vi "Berechnung Limit mbar.vi"(0 "Volumen in mm³":dbl, 1 "t2":timestamp, 2 "t1":timestamp, 7 "p1":sgl, 9 "T2 in C°":sgl, 11 "T1 in C°":sgl, 12 "Fluss in l/min":sgl) -> (4 "Limit in mbar":sgl format="%#.9f", 8 "p2":dbl)   [LabVIEW 2020, in "EPA 1065.lvlib" / "Dichtheitstest 1065-345.lvlib"]
uses:
  Dichtheitstest 1065-345.lvlib
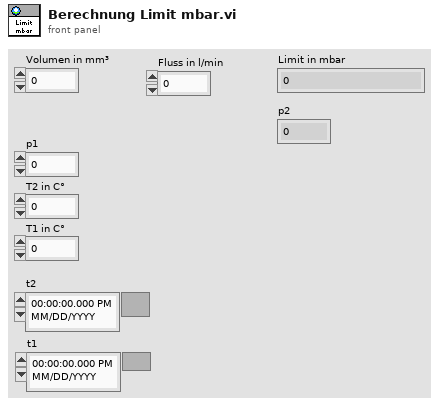
[diagram p1: front panel]
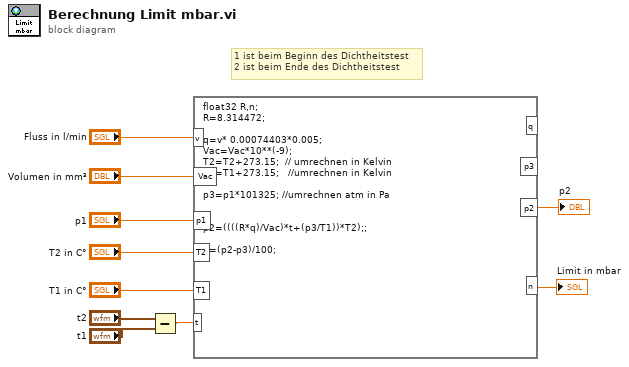
[diagram p0: block diagram]
diagram:
  # "1 ist beim Beginn des Dichtheitstest\n2 ist beim Ende des Dichtheitstest"
  n1 = Subtract(x="t2", y="t1") -> (x-y=w3:dbl)
  n2 = formula code="float32 R,n;\nR=8.314472;\n\nq=v* 0.00074403*0.005;\nVac=Vac*10**(-9);\nT2=T2+273.15;  // umrechnen in Kelvin\nT1=T1+273.15;   //umrechnen in Kelvin\n\np3=p1*101325; //umrechnen atm in Pa\n\n\np2=((((R*q)/Vac)*t+(p3/T1))*T2);;\n\nn=(p2-p3)/100;"("Vac"="Volumen in mm³", "p1"="p1", "T2"="T2 in C°", "T1"="T1 in C°", "t"=w3, "v"="Fluss in l/min") -> ("n"=→"Limit in mbar":sgl, "p2"=→"p2":dbl)  [unwired: 2 out]
